vi "Is Generation Done.vi"(0 "channel status in":T2, 5 "configuration":T1) -> (4 "channel status out":T2)   [LabVIEW 2020, in "GettingStarted_Gen_148X_FPGA.lvlib"]
uses:
  GettingStarted_Gen_148X_FPGA.lvlib
  Types/Serial Output Channel Status.ctl
  Common/Types/DRAM Status.ctl
  Types/Serial Output Channel Datapath Configuration.ctl
  Common/GettingStarted_Common_148X_FPGA.lvlib
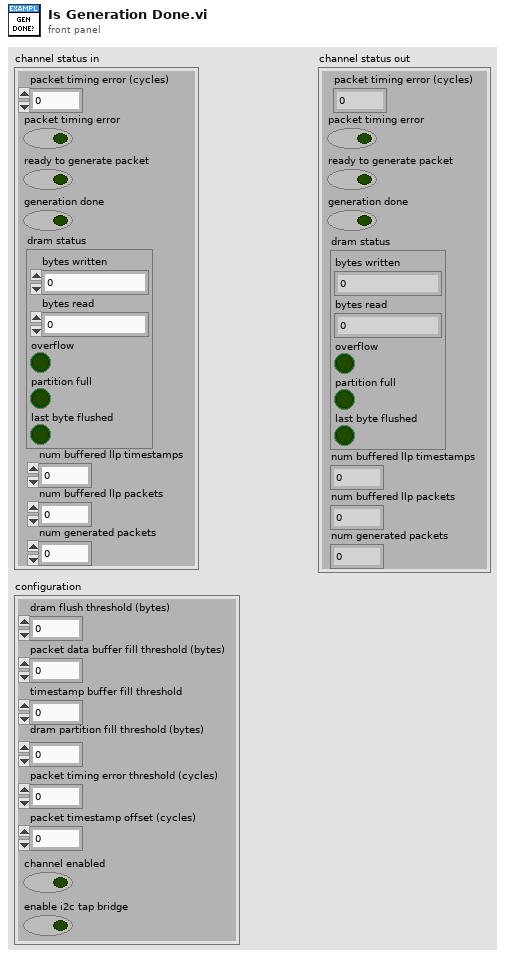
[diagram p1: front panel]
types:
  T1 = typedef "GettingStarted_Gen_148X_FPGA.lvlib/Serial Output Channel Datapath Configuration.ctl" = cluster{"dram flush threshold (bytes)":u64, "packet data buffer fill threshold (bytes)":u64, "timestamp buffer fill threshold":u32, "packet timing error threshold (cycles)":u64, "channel enabled":bool, "dram partition fill threshold (bytes)":u64, "enable i2c tap bridge":bool, "packet timestamp offset (cycles)":i64}
  T2 = typedef "GettingStarted_Gen_148X_FPGA.lvlib/Serial Output Channel Status.ctl" = cluster{"num buffered llp packets":fxp<+,14,14>, "packet timing error (cycles)":u64, "packet timing error":bool, "ready to generate packet":bool, "dram status":T3, "num buffered llp timestamps":u32, "generation done":bool, "num generated packets":u64}
  T3 = typedef "GettingStarted_Common_148X_FPGA.lvlib/DRAM Status.ctl" = cluster{"bytes written":u64, "bytes read":u64, "overflow":bool, "partition full":bool, "last byte flushed":bool}
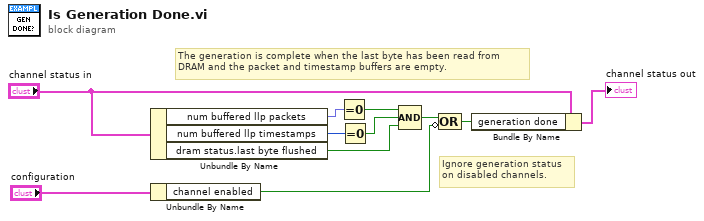
[diagram p0: block diagram]
diagram:
  # "Ignore generation status \non disabled channels."
  # "The generation is complete when the last byte has been read from \nDRAM and the packet and timestamp buffers are empty."
  n1 = Unbundle By Name("channel status in") -> ("num buffered llp packets"=w9:fxp<+,14,14>, "num buffered llp timestamps"=w8:u32, "dram status.last byte flushed"=w1:bool)
  n2 = Unbundle By Name("configuration") -> ("channel enabled"=w2:bool)
  n3 = Equal To 0?(x=w9) -> (x = 0?=w11:bool)
  n4 = Equal To 0?(x=w8) -> (x = 0?=w10:bool)
  n5 = Compound Arithmetic op=AND(w11, w10, w1) -> (w4:bool)
  n6 = Compound Arithmetic op=OR(w4, invert w2) -> (w3:bool)
  n7 = Bundle By Name(cluster="channel status in", "generation done"=w3) -> (→"channel status out":T2)
